vi "myRIO_BRig_RT_dataExp_IblockUntilReward.vi"() -> (2 "output_I_blockUntilReward":i32)   [LabVIEW 2014]
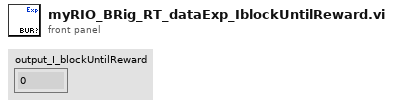
[diagram p1: front panel]
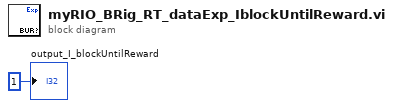
[diagram p0: block diagram]
diagram:
  "output_I_blockUntilReward" <- 1 ("output_iBlock")
